vi "AuMT8852B Event Status Query.vi"(8 "error in (no error)":errorcluster, 11 "VISA session":refnum<visa-resource-name>) -> (0 "error out":errorcluster, 2 "error code":i32, 3 "VISA session out":refnum<visa-resource-name>, 4 "Flags":T1, 6 "Value":i32)   [LabVIEW 2017]
doc: "Anritsu MT8852B Bluetooth Tester\n\nReturns the IEE-488.2 standard Event Status Register.\n\nBit 7 (most significant bit) - Power on - this bit is set on power up of the device only and cleared if the instrument is reset or receives a *CLS command. This bit only indicates that a power on has occurred.\n\nBit 6 - User reqest - unused.\n\nBit 5 - Command error - received an unrecognized command.\n\nBit 4 - Execution error - could not execute a command. For example, a parameter is out of the allowable range.\n\nBit 3 - Device dependent error - the specific error can be found by using the ERRLST command.\n\nBit 2 - Query error.\n\nBit 1 - Request control. GPIB controllers only.\n\nBit 0 (least significant bit) - Operation complete. When a program message that includes the *OPC command has been completed and the GPIB interface is idle with any responses read out of the output buffer, this bit is set. For example, if the last command in a configuration sequence is *OPC, the OPC bit in the event status register will be set when that configuration list has been completed.\n\nOUTPUTS\nFlags - meaning of each individual bit in the register.\nValue - integer value (0-255) of the register."
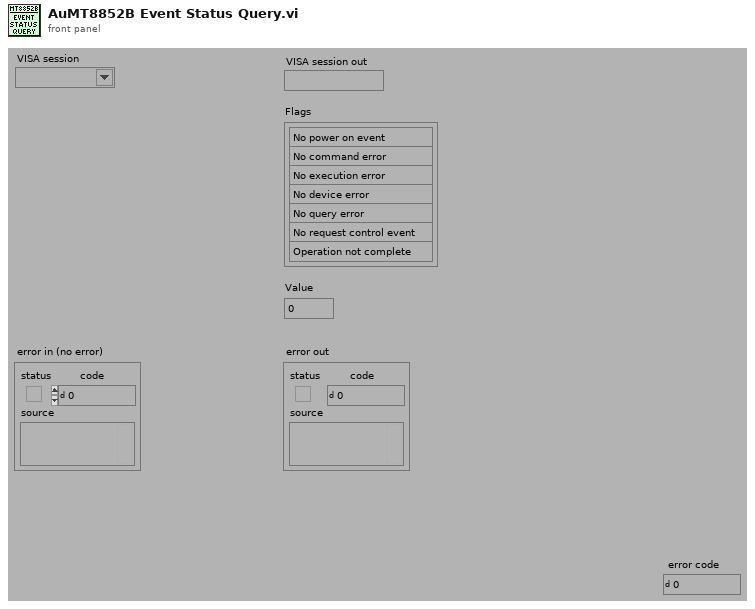
[diagram p1: front panel]
types:
  T1 = cluster{"Power on":enum16{"No power on event", "Power on event"}, "Command":enum16{"No command error", "Command error"}, "Execution":enum16{"No execution error", "Execution error"}, "Device":enum16{"No device error", "Device error"}, "Query":enum16{"No query error", "Query error"}, "Request control":enum16{"No request control event", "Request control event"}, "Operation":enum16{"Operation not complete", "Operation complete"}}
  T2 = enum16{"Simulate", "Range check", "Cache", "Query instrument status"}
  T3 = cluster{"[0]":i16, "[1]":i16, "[2]":i16, "[3]":i16, "[4]":i16, "[5]":i16, "[6]":i16, "[7]":i16}
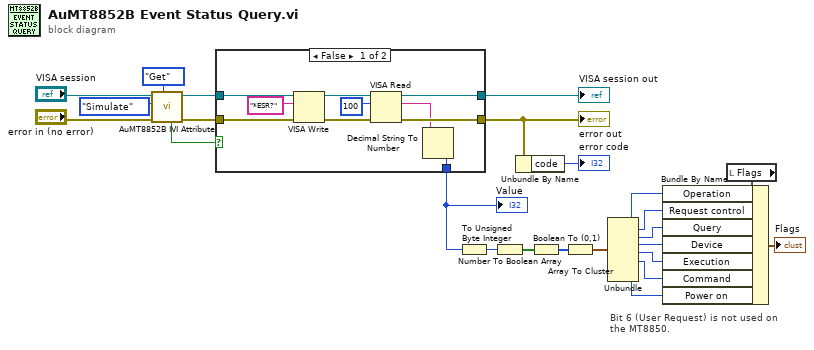
[diagram p0: block diagram]
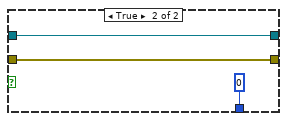
[diagram p2: hidden frame]
diagram:
  # "Bit 6 (User Request) is not used on\nthe MT8850."
  n1 = call <instrlib>:"AuMT8852B IVI Attribute.vi"("Set/Get (Set)"=enum16{"Set", "Get"}."Get", "error in (no error)"="error in (no error)", "Flag (Simulate)"=T2."Simulate", "VISA session"="VISA session") -> ("error out"=w20:errorcluster, "VISA session out"=w21:refnum<visa-resource-name>, "Value out"=w17:bool)  [unwired: 5 in]
  n2 = case shown="False" w17 {
    tunnel: [w28 w36] -> w1
    tunnel: [w29 w37] -> w22
    tunnel: w21 -> [w34 w37]
    tunnel: w20 -> [w33 w36]
    tunnel: [w25 0] -> w16
    frame False {
      n3 = VISA Write(VISA resource name=w34, write buffer="*ESR?" ("write buffer (\"\")"), error in (no error)=w33) -> (VISA resource name out=w31:refnum<visa-resource-name>, error out=w30:errorcluster)  [unwired: 1 out]
      n4 = VISA Read(VISA resource name=w31, byte count=u32 100 ("byte count (0)"), error in (no error)=w30) -> (VISA resource name out=w29:refnum<visa-resource-name>, read buffer=w26:string, error out=w28:errorcluster)  [unwired: 1 out]
      n5 = Decimal String To Number(string=w26) -> (number=w25:i32)  [unwired: 2 in, 1 out]
    }
    frame True {
    }
  }
  "error out" <- w1
  "VISA session out" <- w22
  "Value" <- w16
  n6 = To Unsigned Byte Integer(number=w16) -> (unsigned 8bit integer=w15:u8)
  n7 = Number To Boolean Array(number=w15) -> (Boolean array=w14:bool[])
  n8 = Unbundle By Name(w1) -> ("code"=→"error code":i32)
  n9 = Boolean To (0,1)(Boolean=w14) -> (0, 1=w13:i16[])
  n10 = Array To Cluster(array=w13) -> (cluster=w5:T3)
  n11 = Unbundle(w5) -> ("[0]"=w12:i16, "[1]"=w11:i16, "[2]"=w10:i16, "[3]"=w9:i16, "[4]"=w8:i16, "[5]"=w7:i16, "[7]"=w6:i16)  [unwired: 1 out]
  n12 = local read "Flags"() -> (w4:T1)
  n13 = Bundle By Name(cluster=w4, "Operation"=w12, "Request control"=w11, "Query"=w10, "Device"=w9, "Execution"=w8, "Command"=w7, "Power on"=w6) -> (→"Flags":T1)
